vi "Example Read.vi"() -> ()   [LabVIEW 2010]
uses:
  C:/tf/play/labview/Tinkerforge.dll
  Tinkerforge.dll
panel:
  out "data [hex]":u8[](array[numeric]) format="%x"
  out "identifier [hex]":i64 format="%x"
  out "frameType":u8
  in  "stop":bool
  in  "uid":string="5556"
  in  "port":i32=4223
  in  "host":string="localhost"
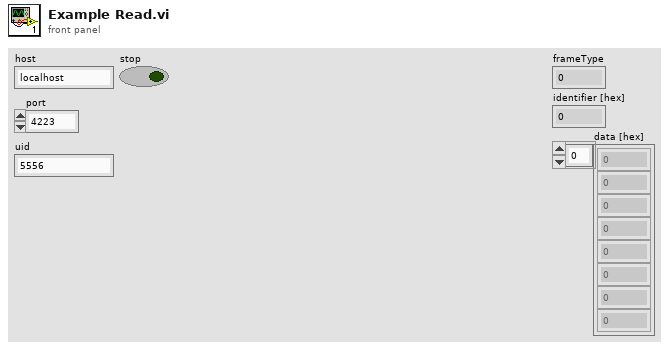
[diagram p1: front panel]
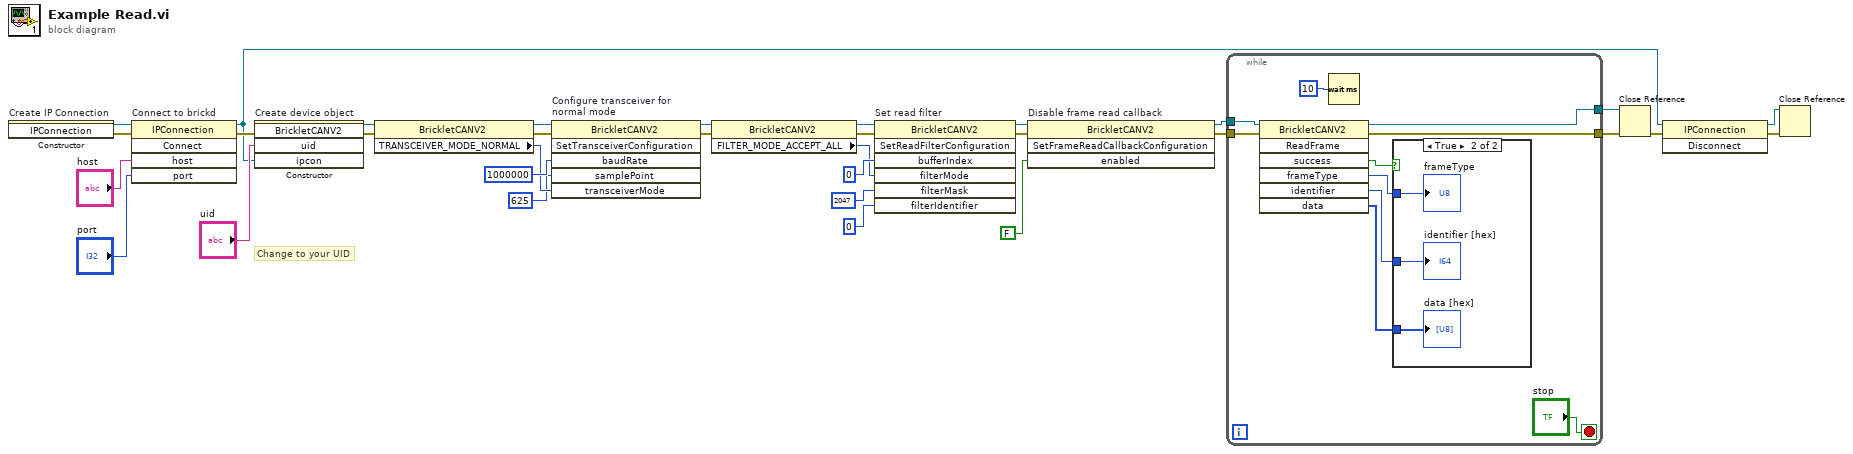
[diagram p0: block diagram]
diagram:
  # "Change to your UID"
  n1 = constructor on="Create IP Connection" class="IPConnection"() -> (reference out=w32:refnum<k24>, error out=w23:errorcluster)  [unwired: 3 in, 1 out]
  n2 = invoke on="Connect to brickd" class="IPConnection" method="Connect"(reference=w32, error in=w23, "host"="host", "port"="port") -> (reference out=w25:refnum<k24>, error out=w28:errorcluster)  [unwired: 1 in, 3 out]
  n3 = constructor on="Create device object" class="BrickletCANV2"(error in=w28, "uid"="uid", "ipcon"=w25) -> (reference out=w21:refnum<k24>, error out=w22:errorcluster)  [unwired: 2 in, 3 out]
  n4 = property class="BrickletCANV2"(reference=w21, error in=w22) -> (reference out=w19:refnum<k24>, error out=w20:errorcluster, "TRANSCEIVER_MODE_NORMAL"=w16:u8)
  n5 = invoke on="Configure transceiver for\nnormal mode" class="BrickletCANV2" method="SetTransceiverConfiguration"(reference=w19, error in=w20, "baudRate"=i64 1000000, "samplePoint"=625, "transceiverMode"=w16) -> (reference out=w2:refnum<k24>, error out=w3:errorcluster)  [unwired: 1 in, 4 out]
  n6 = property class="BrickletCANV2"(reference=w2, error in=w3) -> (reference out=w1:refnum<k24>, error out=w4:errorcluster, "FILTER_MODE_ACCEPT_ALL"=w7:u8)
  n7 = invoke on="Set read filter" class="BrickletCANV2" method="SetReadFilterConfiguration"(reference=w1, error in=w4, "bufferIndex"=u8 0, "filterMode"=w7, "filterMask"=i64 2047, "filterIdentifier"=i64 0) -> (reference out=w9:refnum<k24>, error out=w10:errorcluster)  [unwired: 1 in, 5 out]
  n8 = invoke on="Disable frame read callback" class="BrickletCANV2" method="SetFrameReadCallbackConfiguration"(reference=w9, error in=w10, "enabled"=FALSE) -> (reference out=w12:refnum<k24>, error out=w13:errorcluster)  [unwired: 1 in, 2 out]
  n9 = while {
    tunnel: [w41] -> w14
    tunnel: w13 -> [w42]
    tunnel: w12 -> [w40]
    tunnel: [w39] -> w11
    stop <- "stop" stop-if-true
    n10 = invoke class="BrickletCANV2" method="ReadFrame"(reference=w40, error in=w42) -> (reference out=w39:refnum<k24>, error out=w41:errorcluster, "success"=w37:bool, "frameType"=w36:u8, "identifier"=w35:i64, "data"=w34:u8[])  [unwired: 5 in, 1 out]
    n11 = Wait (ms)(milliseconds to wait=u32 10) -> ()  [unwired: 1 out]
    n12 = case shown="True" w37 {
      tunnel: w36 -> [_ w45]
      tunnel: w35 -> [_ w44]
      tunnel: w34 -> [_ w43]
      frame False {
      }
      frame True {
        "frameType" <- w45
        "data [hex]" <- w43
        "identifier [hex]" <- w44
      }
    }
  }
  n13 = Close Reference(reference=w11, error in (no error)=w14) -> (error out=w27:errorcluster)
  n14 = invoke class="IPConnection" method="Disconnect"(reference=w25, error in=w27) -> (reference out=w24:refnum<k24>, error out=w26:errorcluster)  [unwired: 1 in, 1 out]
  n15 = Close Reference(reference=w24, error in (no error)=w26) -> ()  [unwired: 1 out]
